vi "Convert Hex String to Array.vi"(7 "Hex String In":string) -> (8 "Hex Array Out":u8[](array[numeric]) format="%.0x", 10 "Hex Array Out":string[](array[string]))   [LabVIEW 2014, in "GEA2_Toolkit.lvlib"]
uses:
  library/GEA2_Toolkit.lvlib
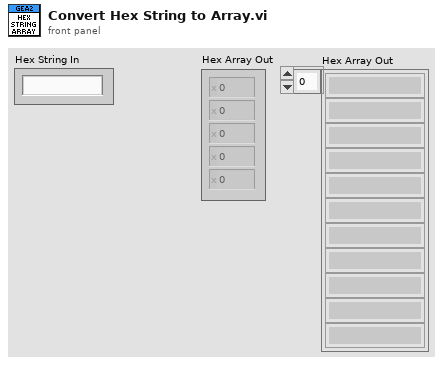
[diagram p1: front panel]
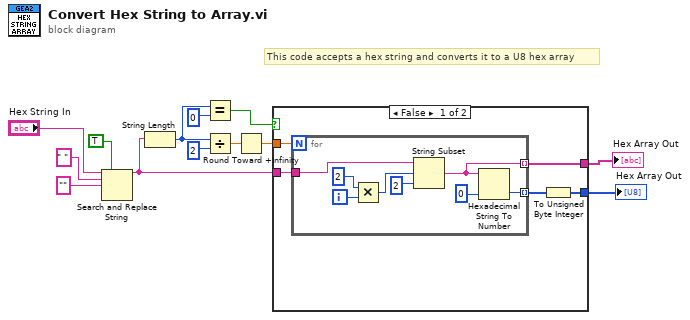
[diagram p0: block diagram]
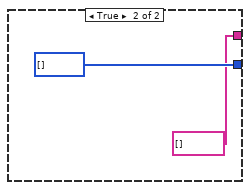
[diagram p2: hidden frame]
diagram:
  # "This code accepts a hex string and converts it to a U8 hex array"
  n1 = Search and Replace String(replace all?=TRUE ("replace all? (F)"), input string="Hex String In", search string=" ", replace string="" ("replace string (\"\")")) -> (result string=w11:string)  [unwired: 4 in, 3 out]
  n2 = String Length(string=w11) -> (length=w7:i32)
  n3 = Equal?(x=w7, y=0) -> (x = y?=w9:bool)
  n4 = Divide(x=w7, y=2) -> (x/y=w4:dbl)
  n5 = Round Toward +Infinity(x=w4) -> (ceil(x): smallest int >= x=w5:dbl)
  n6 = case shown="False" w9 {
    tunnel: w11 -> [w18 _]
    tunnel: [w17 u8[] []] -> w2
    tunnel: w5 -> [w16 _]
    tunnel: [w14 string[] []] -> w1
    frame False {
      n7 = for {
        N: w16 -> [_]
        tunnel: w18 -> [w24]
        tunnel: [w20] -> w15 mode=indexing
        tunnel: [w19] -> w14 mode=indexing
        i -> [w26]
        n8 = Multiply(x=2, y=w26) -> (x*y=w23:i32)
        n9 = String Subset(string=w24, offset (0)=w23, length (rest)=2 ("length (rest)")) -> (substring=w19:string)
        n10 = Hexadecimal String To Number(string=w19, default (0uL)=u32 0 ("default (0 U32)")) -> (number=w20:u32)  [unwired: 1 in, 1 out]
      }
      n11 = To Unsigned Byte Integer(number=w15) -> (unsigned 8bit integer=w17:u8[])
    }
    frame True {
    }
  }
  "Hex Array Out" <- w2
  "Hex Array Out" <- w1
